vi "Get Panel Valid VI Refnum.vi"(8 "error in (no error)":errorcluster, 11 "EditPanel API in":refnum<class "EditPanel API.lvclass">) -> (0 "error out":errorcluster, 2 "VI Running Refnum":refnum<vi>, 3 "EditPanel API out":refnum<class "EditPanel API.lvclass">)   [LabVIEW 2015, in "EditPanel API.lvlib" / "EditPanel API.lvclass"]
uses:
  EditPanel API.lvclass
  EditPanel API.lvclass/EditPanel API.ctl
  Console Reply/Console Reply/Console Reply.lvclass/Console Reply.ctl
  Console Reply/Console Reply/Console Reply.lvclass
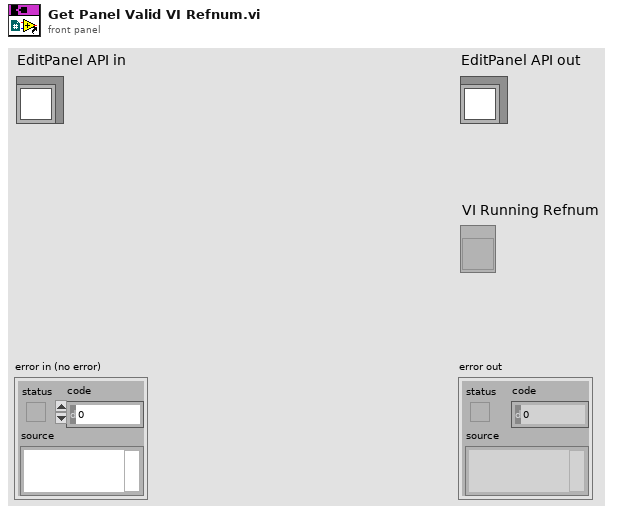
[diagram p1: front panel]
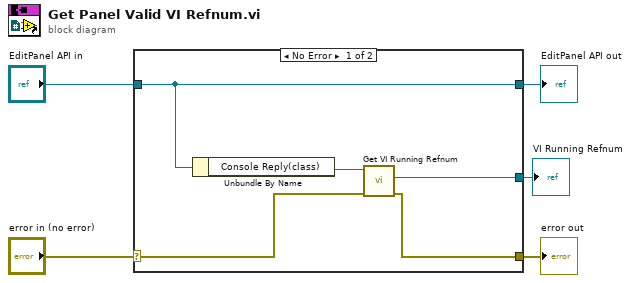
[diagram p0: block diagram]
diagram:
  n1 = case shown="No Error" "error in (no error)" {
    selector: "error in (no error)" -> [w8 w11]
    tunnel: [w6 w11] -> w4
    tunnel: [w10 w12] -> w2
    tunnel: "EditPanel API in" -> [w10 w12]
    tunnel: [w7 _] -> w1
    frame No Error {
      n2 = Unbundle By Name(w10) -> ("Console Reply(class)"=w9:refnum<class "Console Reply.lvclass">)
      n3 = call "Get VI Running Refnum.vi"("error in (no error)"=w8, "Console Reply.lvclass"=w9) -> ("error out"=w6:errorcluster, "VI Running Refnum"=w7:refnum<vi>)  [unwired: 7 in, 1 out]
    }
    frame Error {
    }
  }
  "error out" <- w4
  "EditPanel API out" <- w2
  "VI Running Refnum" <- w1
